vi "SelectAuxValueInput.vi"(8 "error in (no error)":errorcluster, 9 "Aux box input selection":bool caption="Aux input selection toggle", 10 "Aux code input":i32 min=0 max=255 step=1, 11 "Aux box input":i32[](listbox)) -> (0 "error out":errorcluster, 3 "aux decimal integer string":string)   [LabVIEW 2023, in "Thermotron 8800.lvlib"]
uses:
  Thermotron 8800.lvlib
panel:
  # "Aux box input selection"
  # "Aux code input selection"
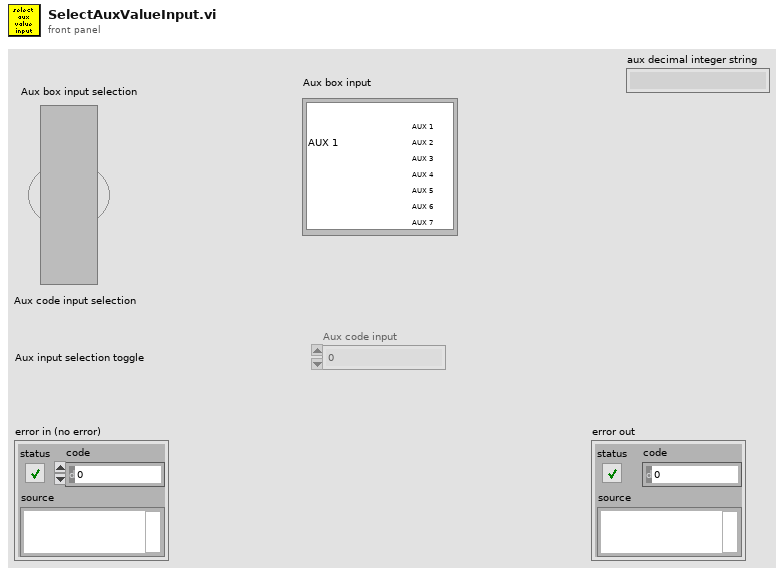
[diagram p1: front panel]
types:
  T1 = enum8{"Enabled", "Disabled", "Disabled and Grayed Out"}
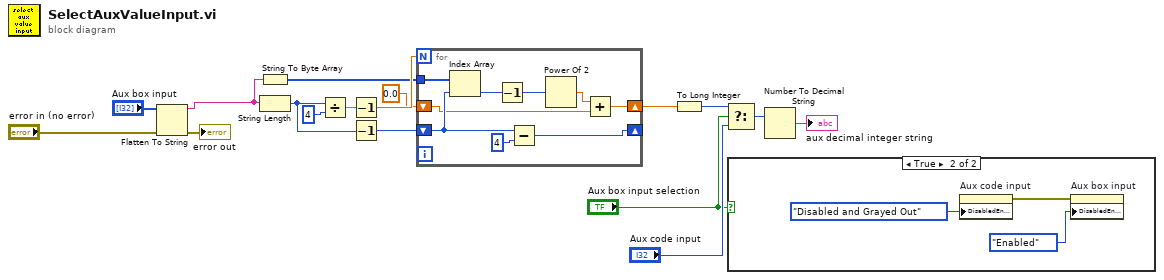
[diagram p0: block diagram]
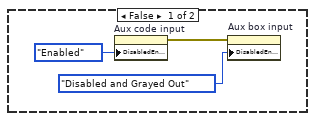
[diagram p2: hidden frame]
diagram:
  n1 = Flatten To String(anything="Aux box input", error in (no error)="error in (no error)") -> (data string=w17:string, error out=→"error out":errorcluster)  [unwired: 2 in, 1 out]
  n2 = String To Byte Array(string=w17) -> (unsigned byte array=w12:u8[])
  n3 = String Length(string=w17) -> (length=w13:i32)
  n4 = Divide(x=w13, y=4) -> (x/y=w15:dbl)
  n5 = Decrement(x=w15) -> (x-1=w14:dbl)
  n6 = Decrement(x=w13) -> (x-1=w11:i32)
  n7 = for {
    N: w14 -> [_]
    tunnel: w12 -> [w26]
    shift-right: [w23] -> _
    shift-left: w11 -> [w25]
    shift-right: [w18] -> w6
    shift-left: 0.0 -> [w19]
    n8 = Index Array(array=w26, index=w25) -> (element=w22:u8)
    n9 = Decrement(x=w22) -> (x-1=w21:u8)
    n10 = Subtract(x=w25, y=4) -> (x-y=w23:i32)
    n11 = Power Of 2(x=w21) -> (2^x=w20:dbl)
    n12 = Add(x=w20, y=w19) -> (x+y=w18:dbl)
  }
  n13 = To Long Integer(number=w6) -> (32bit integer=w7:i32)
  n14 = Select(t=w7, s="Aux box input selection", f="Aux code input") -> (s? t:f=w5:i32)
  n15 = case shown="True" "Aux box input selection" {
    frame False {
      n16 = property on="Aux code input" class="DigNum (strict)"("DisabledEnum"=T1."Enabled" ("Disabled")) -> (error out=w27:errorcluster)  [unwired: 2 in, 1 out]
      n17 = property on="Aux box input" class="LstBox (strict)"(error in=w27, "DisabledEnum"=T1."Disabled and Grayed Out" ("Disabled")) -> ()  [unwired: 1 in, 2 out]
    }
    frame True {
      n18 = property on="Aux code input" class="DigNum (strict)"("DisabledEnum"=T1."Disabled and Grayed Out" ("Disabled")) -> (error out=w31:errorcluster)  [unwired: 2 in, 1 out]
      n19 = property on="Aux box input" class="LstBox (strict)"(error in=w31, "DisabledEnum"=T1."Enabled" ("Disabled")) -> ()  [unwired: 1 in, 2 out]
    }
  }
  n20 = Number To Decimal String(number=w5) -> (decimal integer string=→"aux decimal integer string":string)  [unwired: 1 in]
